vi "Read Configuration Parameters.vi"(8 "error in (no error)":errorcluster, 10 "refnum":T1, 11 "monitor configuration in":refnum<class "CCD monitor configuration.lvclass">) -> (0 "error out":errorcluster, 2 "refnum out":T1, 3 "monitor configuration out":refnum<class "CCD monitor configuration.lvclass">)   [LabVIEW 2016, in "CCD monitor.lvlib" / "CCD monitor configuration.lvclass"]
uses:
  <userlib>/Common Components/Hardware/Abstract System/Monitor/CCD monitor configuration.lvclass
  <vilib>/Utility/config.llb/Config Data RefNum.ctl
  <userlib>/Common Components/Hardware/Abstract System/Monitor/CCD monitor configuration.lvclass/CCD monitor configuration.ctl
  <userlib>/Common Components/Hardware/CCD/CCD Configuration.lvclass/CCD Configuration.ctl
  <userlib>/Common Components/Hardware/Abstract System/Monitor/CCD monitor.lvclass/CCD monitor.ctl
  <userlib>/Common Components/Hardware/CCD/CCD/CCD.lvclass
  <userlib>/Common Components/Hardware/Abstract System/Monitor/CCD monitor.lvclass
  <userlib>/Common Components/Hardware/CCD/CCD Configuration.lvclass
  <vilib>/Utility/config.llb/NI_LVConfig.lvlib
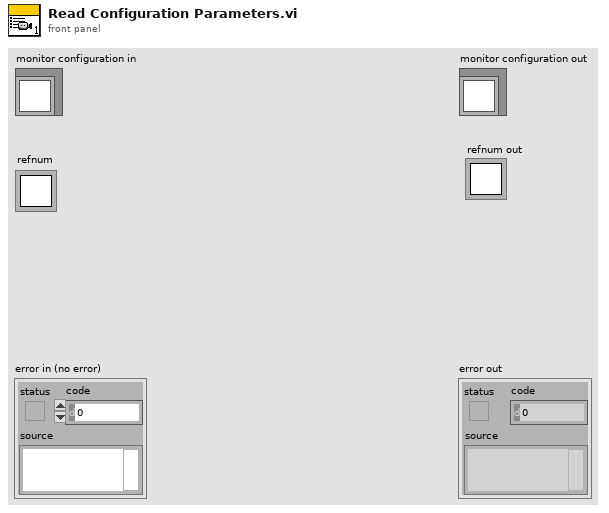
[diagram p1: front panel]
types:
  T1 = typedef "NI_LVConfig.lvlib/Config Data RefNum.ctl" = refnum<k1>
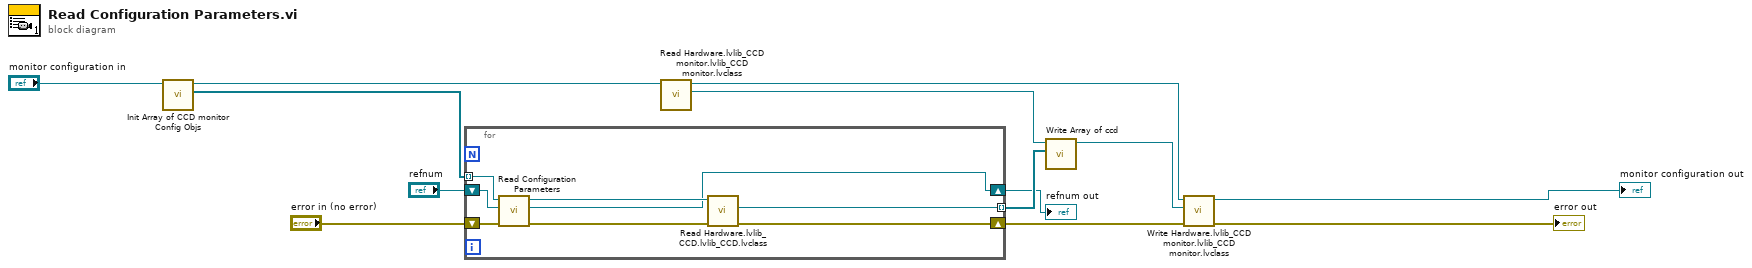
[diagram p0: block diagram]
diagram:
  n1 = call <userlib>:"Init Array of CCD monitor Config Objs.vi"("Hardware.lvlib:CCD monitor.lvlib:CCD monitor configuration.lvclass"="monitor configuration in") -> ("Array of CCD monitor"=w12:refnum<class "CCD Configuration.lvclass">[], "reference out"=w8:refnum<class "CCD monitor configuration.lvclass">)  [unwired: 8 in, 1 out]
  n2 = for {
    tunnel: w12 -> [w21] mode=indexing
    shift-right: [w14] -> w1
    shift-left: "refnum" -> [w20]
    shift-right: [w16] -> w3
    shift-left: "error in (no error)" -> [w19]
    tunnel: [w17] -> w9 mode=indexing
    n3 = call-dynamic "Read Configuration Parameters.vi"("error in (no error)"=w19, "refnum"=w20, "CCD Configuration in"=w21) -> ("error out"=w15:errorcluster, "refnum out"=w14:T1, "CCD Configuration out"=w18:refnum<class "CCD Configuration.lvclass">)  [unwired: 6 in]
    n4 = call <userlib>:"Read Hardware.lvlib_CCD.lvlib_CCD.lvclass.vi"("error in (no error)"=w15, "CCD Configuration in"=w18) -> ("error out"=w16:errorcluster, "Hardware.lvlib:CCD.lvlib:CCD.lvclass"=w17:refnum<class "CCD.lvclass">)  [unwired: 7 in, 1 out]
  }
  "refnum out" <- w1
  n5 = call <userlib>:"Read Hardware.lvlib_CCD monitor.lvlib_CCD monitor.lvclass.vi"("CCD monitor configuration in"=w8) -> ("Hardware.lvlib:CCD monitor.lvlib:CCD monitor.lvclass"=w7:refnum<class "CCD monitor.lvclass">, "CCD monitor configuration out"=w6:refnum<class "CCD monitor configuration.lvclass">)  [unwired: 8 in, 1 out]
  n6 = call <userlib>:"Write Array of ccd.vi"("Array of ccd"=w9, "CCD monitor in"=w7) -> ("CCD monitor out"=w5:refnum<class "CCD monitor.lvclass">)  [unwired: 9 in]
  n7 = call <userlib>:"Write Hardware.lvlib_CCD monitor.lvlib_CCD monitor.lvclass.vi"("error in (no error)"=w3, "Hardware.lvlib:CCD monitor.lvlib:CCD monitor.lvclass"=w5, "CCD monitor configuration in"=w6) -> ("error out"=→"error out":errorcluster, "CCD monitor configuration out"=→"monitor configuration out":refnum<class "CCD monitor configuration.lvclass">)  [unwired: 7 in]
